vi "GetHighPrioritySensors.vi"   [LabVIEW 2019]
doc: "All high priority sensor reads and safety interlock calculations should be placed in this VI."
uses:
  sensors.vi
  dsdata.vi
  <vilib>/Rock Robotics/WPI/DriverStation/WPI_DriverStationRobotMode2.ctl
  outputs.vi
  refnums.vi
  GRNF_CTREMotor.vi
  <vilib>/Rock Robotics/WPI/ThirdParty/Phoenix-LabVIEW/Motor Controller/Get/CTRE_Phoenix_MotorController_GetSelectedSensorData.vi
  dscommands.vi
  GRNF_DIC.vi
types:
  T1 = typedef "WPI_DriverStationRobotMode2.ctl" = enum16{"Autonomous Disabled", "Autonomous Enabled", "Teleop Disabled", "Teleop Enabled", "Disconnected", "Finish", "Test Disabled", "Test Enabled", "Emergency Stopped"}
  T2 = enum16{"Low Gear", "High Gear", "Transiting", "Unknown", "Force Low Gear"}
  T3 = typedef "WPI_CounterDevRef.ctl" = cluster{"DevStatus":errorcluster, "CntIndex":T4}
  T4 = typedef "FPGA_CounterCtrSystemIndex.ctl" = enum8{"Ctr 0", "Ctr 1", "Ctr 2", "Ctr 3", "Ctr 4", "Ctr 5", "Ctr 6", "Ctr 7", "Invalid"}
  T5 = typedef "WPI_MotorControlDeviceRef.ctl" = cluster{"DeviceStatus":errorcluster, "Type":T6, "PWM":cluster{"PWM Channel":T7, "DeadBand":T8}, "CAN":cluster{"Device Number":u8, "SetOutput VI Ref":variant, "GetOutput VI Ref":variant, "Enable VI Ref":variant, "Disable VI Ref":variant, "Data":variant}, "Invert":bool, "DIO PWM":cluster{"PWM \"Enable\" Channel":T7, "DIOChannel":T9, "PWM Rate":dbl}}
  T6 = typedef "WPI_MotorControlType.ctl" = enum16{"PWM", "CAN", "DIO PWM"}
  T7 = typedef "FPGA_DIOPWMChannel.ctl" = enum8{"PWM 0", "PWM 1", "PWM 2", "PWM 3", "PWM 4", "PWM 5", "PWM 6", "PWM 7", "PWM 8", "PWM 9", "PWM MXP 0", "PWM MXP 1", "PWM MXP 2", "PWM MXP 3", "PWM MXP 4", "PWM MXP 5", "PWM MXP 6", "PWM MXP 7", "PWM MXP 8", "PWM MXP 9", "Invalid"}
  T8 = typedef "WPI_PWMDeadband.ctl" = cluster{"Name":string, "maxPositivePwm":i32, "minPositivePwm":i32, "centerPwm":i32, "maxNegativePwm":i32, "minNegativePwm":i32, "angularRange":u16}
  T9 = typedef "FPGA_DIOChannel.ctl" = enum8{"DIO 0", "DIO 1", "DIO 2", "DIO 3", "DIO 4", "DIO 5", "DIO 6", "DIO 7", "DIO 8", "DIO 9", "DIO MXP 0", "DIO MXP 1", "DIO MXP 2", "DIO MXP 3", "DIO MXP 4", "DIO MXP 5", "DIO MXP 6", "DIO MXP 7", "DIO MXP 8", "DIO MXP 9", "DIO MXP 10", "DIO MXP 11", "DIO MXP 12", "DIO MXP 13", "DIO MXP 14", "DIO MXP 15", "SPI Port CS1", "SPI Port CS2", "SPI Port CS3", "SPI Port MISO", "SPI Port MOSI", "Invalid"}
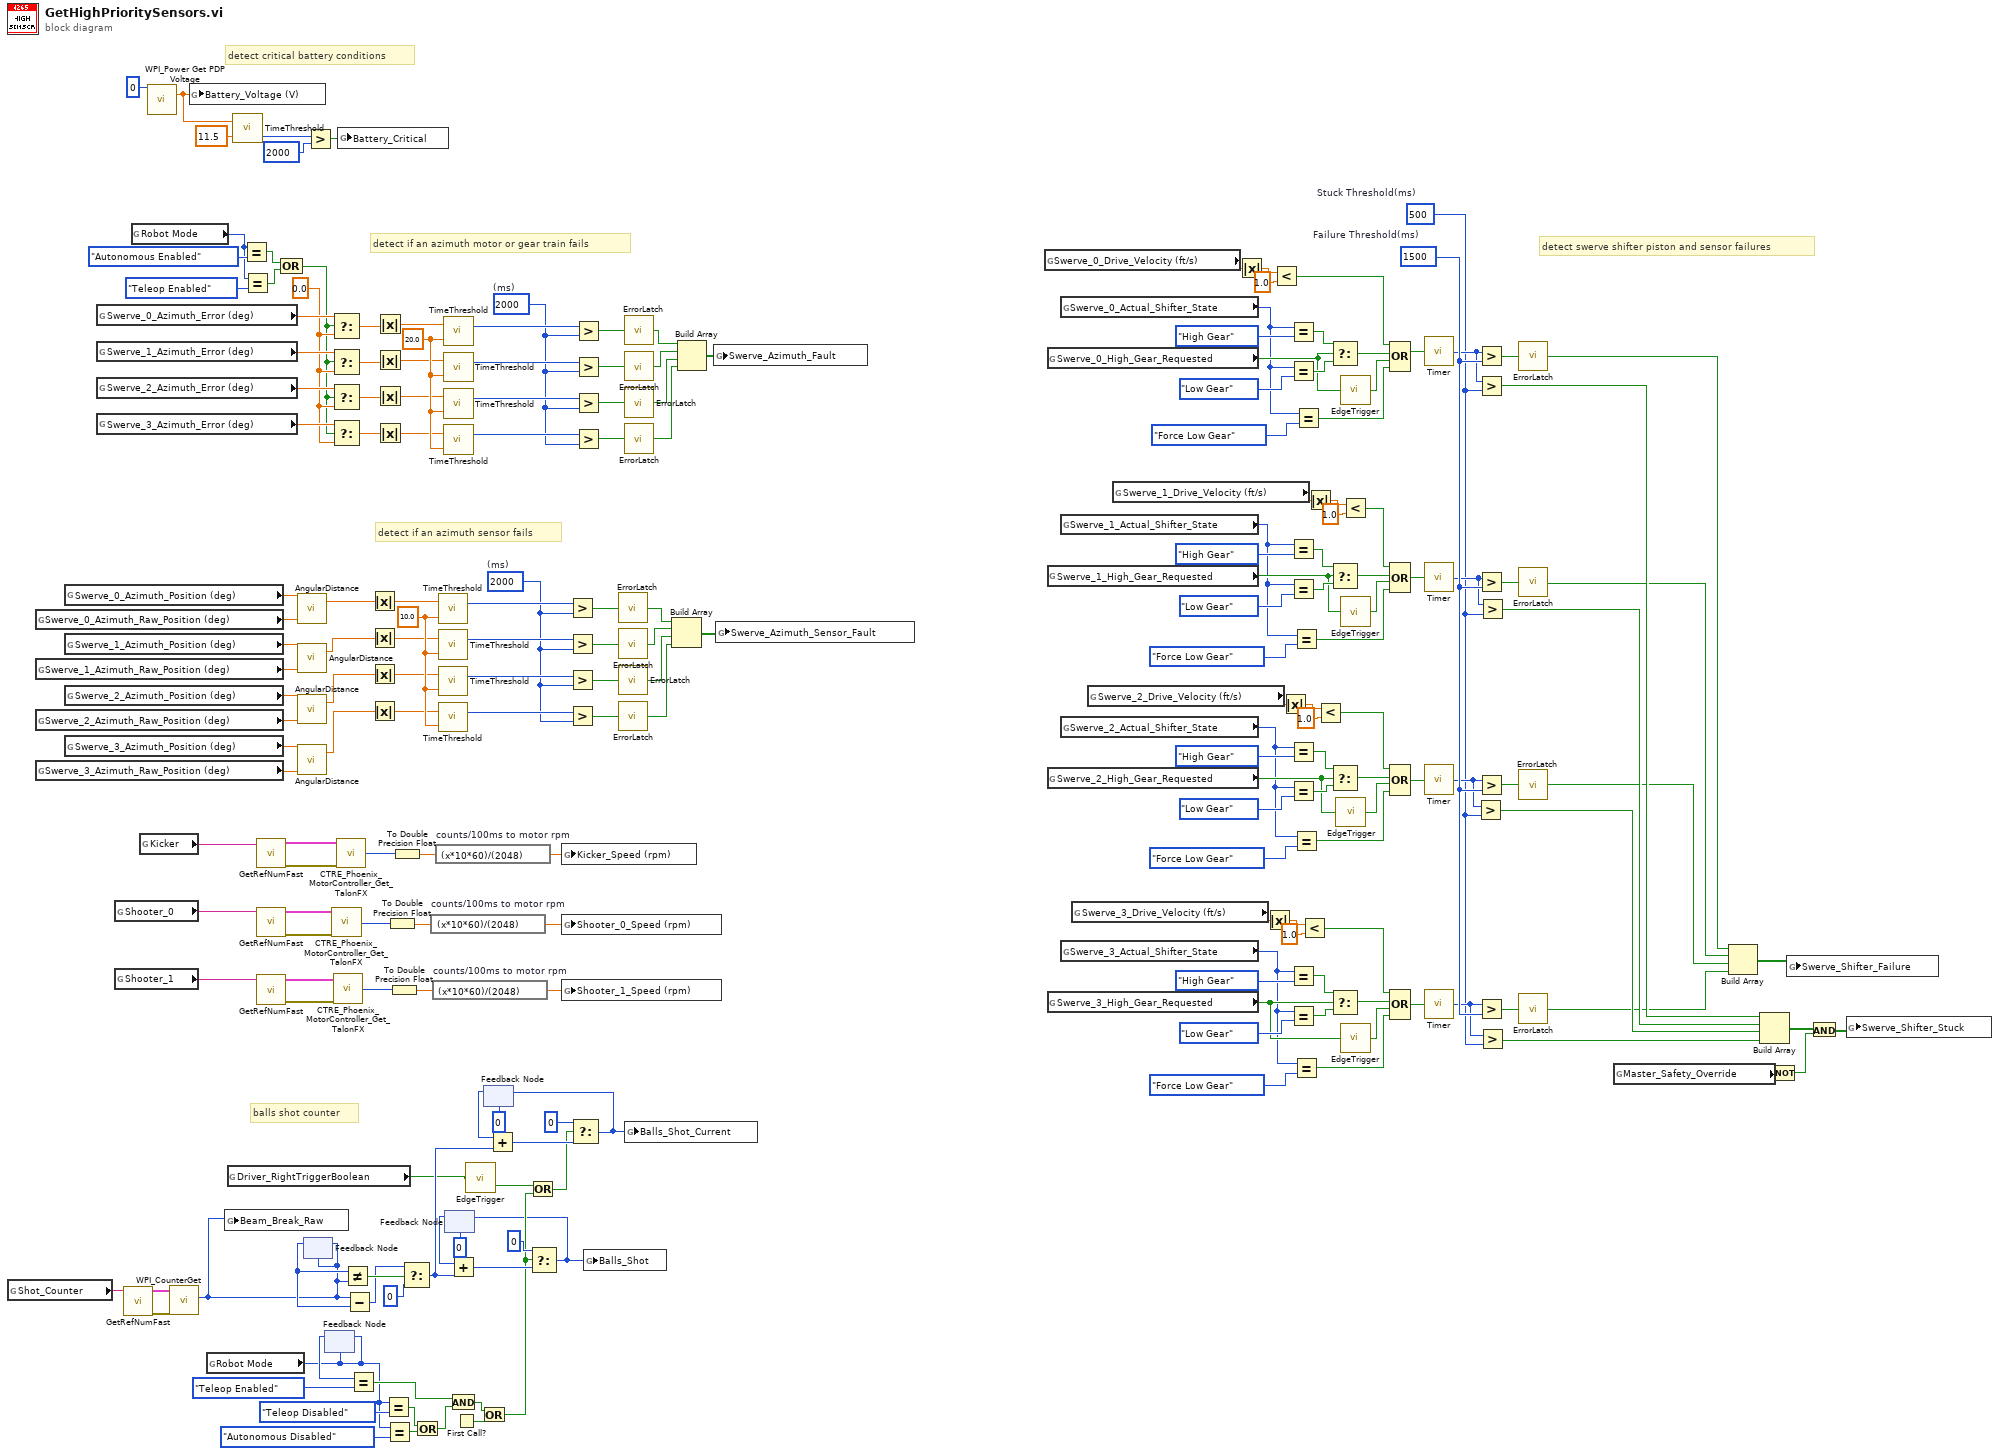
[diagram p0: block diagram]
diagram:
  w99 = u32 500  # Stuck Threshold(ms)
  w124 = u32 2000  # (ms)
  w123 = 10.0 ("Threshold")
  w147 = u32 1500  # Failure Threshold(ms)
  w173 = 0.0
  w196 = u32 2000  # (ms)
  w195 = 20.0 ("Threshold")
  # "balls shot counter"
  # "detect if an azimuth sensor fails"
  # "detect critical battery conditions"
  # "detect swerve shifter piston and sensor failures"
  # "detect if an azimuth motor or gear train fails"
  n1 = global read "refnums.vi" "Shot_Counter"() -> (w15:string)
  n2 = global read "sensors.vi" "Swerve_0_Azimuth_Raw_Position (deg)"() -> (w129:dbl)
  n3 = global read "sensors.vi" "Swerve_1_Azimuth_Raw_Position (deg)"() -> (w108:dbl)
  n4 = global read "sensors.vi" "Swerve_2_Azimuth_Raw_Position (deg)"() -> (w106:dbl)
  n5 = global read "sensors.vi" "Swerve_3_Azimuth_Raw_Position (deg)"() -> (w104:dbl)
  n6 = global read "sensors.vi" "Swerve_0_Azimuth_Position (deg)"() -> (w130:dbl)
  n7 = global read "sensors.vi" "Swerve_1_Azimuth_Position (deg)"() -> (w109:dbl)
  n8 = global read "sensors.vi" "Swerve_2_Azimuth_Position (deg)"() -> (w107:dbl)
  n9 = global read "sensors.vi" "Swerve_3_Azimuth_Position (deg)"() -> (w105:dbl)
  n10 = global read "outputs.vi" "Swerve_0_Azimuth_Error (deg)"() -> (w177:dbl)
  n11 = global read "outputs.vi" "Swerve_1_Azimuth_Error (deg)"() -> (w176:dbl)
  n12 = global read "outputs.vi" "Swerve_2_Azimuth_Error (deg)"() -> (w175:dbl)
  n13 = global read "outputs.vi" "Swerve_3_Azimuth_Error (deg)"() -> (w174:dbl)
  n14 = global read "refnums.vi" "Shooter_0"() -> (w63:string)
  n15 = global read "refnums.vi" "Shooter_1"() -> (w62:string)
  n16 = call-poly "GetRefNumFast.vi"("RefNum Name"=w15) -> ("Error"=w16:errorcluster, "Device Reference"=w17:T3)  [unwired: 5 in]
  n17 = global read "dsdata.vi" "Robot Mode"() -> (w188:T1)
  n18 = global read "refnums.vi" "Kicker"() -> (w64:string)
  n19 = call <vilib>:"WPI_Power Get PDP Voltage.vi"("Power Distribution Panel (0)"=u8 0) -> ("voltage (V)"=w205:dbl)  [unwired: 13 in, 1 out]
  n20 = call <vilib>:"WPI_CounterGet.vi"("error in (no error)"=w16, "CounterDevRef in"=w17) -> ("Value"=w9:i32)  [unwired: 4 in, 5 out]
  n21 = global write "sensors.vi" "Battery_Voltage (V)"(w205) -> ()
  n22 = global read "dsdata.vi" "Robot Mode"() -> (w12:T1)
  n23 = global write "sensors.vi" "Beam_Break_Raw"(w9) -> ()
  n24 = global read "dscommands.vi" "Driver_RightTriggerBoolean"() -> (w13:bool)
  n25 = call "TimeThreshold.vi"("Threshold"=11.5, "Current Value"=w205) -> ("Time Below Threshold (ms)"=w203:u32)  [unwired: 1 out]
  n26 = Equal?(x=w188, y=WPI_DriverStationRobotMode2."Autonomous Enabled") -> (x = y?=w187:bool)
  n27 = Equal?(x=w188, y=WPI_DriverStationRobotMode2."Teleop Enabled") -> (x = y?=w186:bool)
  n28 = call-poly "GetRefNumFast.vi"("RefNum Name"=w64) -> ("Error"=w55:errorcluster, "Device Reference"=w56:T5)  [unwired: 5 in]
  n29 = call-poly "GetRefNumFast.vi"("RefNum Name"=w63) -> ("Error"=w47:errorcluster, "Device Reference"=w48:T5)  [unwired: 5 in]
  n30 = call-poly "GetRefNumFast.vi"("RefNum Name"=w62) -> ("Error"=w45:errorcluster, "Device Reference"=w46:T5)  [unwired: 5 in]
  n31 = Compound Arithmetic op=OR(w187, w186) -> (w168:bool)
  n32 = call "AngularDistance.vi"("Goal Angle (deg) [0,360]"=w129, "Current Angle (deg) [-Inf,+Inf]"=w130) -> ("Signed Angular Distance (deg) [-180,+180]"=w61:dbl)  [unwired: 1 out]
  n33 = call "AngularDistance.vi"("Goal Angle (deg) [0,360]"=w108, "Current Angle (deg) [-Inf,+Inf]"=w109) -> ("Signed Angular Distance (deg) [-180,+180]"=w60:dbl)  [unwired: 1 out]
  n34 = call "AngularDistance.vi"("Goal Angle (deg) [0,360]"=w106, "Current Angle (deg) [-Inf,+Inf]"=w107) -> ("Signed Angular Distance (deg) [-180,+180]"=w59:dbl)  [unwired: 1 out]
  n35 = call "AngularDistance.vi"("Goal Angle (deg) [0,360]"=w104, "Current Angle (deg) [-Inf,+Inf]"=w105) -> ("Signed Angular Distance (deg) [-180,+180]"=w58:dbl)  [unwired: 1 out]
  n36 = feedback #1(w9) -> (w42:i32)
  n37 = feedback-in #1(w9) -> ()
  n38 = Greater?(x=w203, y=u32 2000) -> (0:w201:bool)
  n39 = feedback #2(w12) -> (w32:T1)
  n40 = feedback-in #2(w12) -> ()
  n41 = Select(t=w177, s=w168, f=w173) -> (s? t:f=w172:dbl)
  n42 = Select(t=w176, s=w168, f=w173) -> (s? t:f=w171:dbl)
  n43 = Select(t=w175, s=w168, f=w173) -> (s? t:f=w170:dbl)
  n44 = Select(t=w174, s=w168, f=w173) -> (s? t:f=w169:dbl)
  n45 = call-poly <vilib>:"CTRE_Phoenix_MotorController_Get_TalonFX.vi"("PhoenixMotorControlDevRef"=w48, "error in"=w47) -> ("Velocity (Raw Sensor Units per 100 ms)"=w51:i32)  [unwired: 10 in, 3 out]
  n46 = call-poly <vilib>:"CTRE_Phoenix_MotorController_Get_TalonFX.vi"("PhoenixMotorControlDevRef"=w46, "error in"=w45) -> ("Velocity (Raw Sensor Units per 100 ms)"=w49:i32)  [unwired: 10 in, 3 out]
  n47 = call-poly <vilib>:"CTRE_Phoenix_MotorController_Get_TalonFX.vi"("PhoenixMotorControlDevRef"=w56, "error in"=w55) -> ("Velocity (Raw Sensor Units per 100 ms)"=w53:i32)  [unwired: 10 in, 3 out]
  n48 = global write "sensors.vi" "Battery_Critical"(w201) -> ()
  n49 = Not Equal?(x=w42, y=w9) -> (x != y?=w41:bool)
  n50 = Subtract(x=w9, y=w42) -> (x-y=w40:i32)
  n51 = Equal?(x=w32, y=WPI_DriverStationRobotMode2."Teleop Enabled") -> (x = y?=w31:bool)
  n52 = Absolute Value(x=w61) -> (abs(x)=w122:dbl)
  n53 = Absolute Value(x=w60) -> (abs(x)=w121:dbl)
  n54 = Absolute Value(x=w59) -> (abs(x)=w120:dbl)
  n55 = Absolute Value(x=w58) -> (abs(x)=w119:dbl)
  n56 = Absolute Value(x=w172) -> (abs(x)=w194:dbl)
  n57 = Absolute Value(x=w171) -> (abs(x)=w193:dbl)
  n58 = Absolute Value(x=w170) -> (abs(x)=w192:dbl)
  n59 = Absolute Value(x=w169) -> (abs(x)=w191:dbl)
  n60 = Equal?(x=w12, y=WPI_DriverStationRobotMode2."Teleop Disabled") -> (x = y?=w22:bool)
  n61 = Equal?(x=w12, y=WPI_DriverStationRobotMode2."Autonomous Disabled") -> (x = y?=w23:bool)
  n62 = To Double Precision Float(number=w51) -> (double precision float=w52:dbl)
  n63 = To Double Precision Float(number=w49) -> (double precision float=w50:dbl)
  n64 = To Double Precision Float(number=w53) -> (double precision float=w57:dbl)
  n65 = Select(t=w40, s=w41, f=0) -> (s? t:f=w26:i32)
  n66 = Or(x=w22, y=w23) -> (x .or. y?=w21:bool)
  n67 = expression code="(x*10*60)/(2048)" "counts/100ms to motor rpm"(w52) -> (w44:dbl)
  n68 = expression code="(x*10*60)/(2048)" "counts/100ms to motor rpm"(w50) -> (w43:dbl)
  n69 = expression code="(x*10*60)/(2048)" "counts/100ms to motor rpm"(w57) -> (w54:dbl)
  n70 = call "TimeThreshold.vi"("Threshold"=w123, "Current Value"=w122) -> ("Time Above Threshold (ms)"=w128:u32)  [unwired: 1 out]
  n71 = call "TimeThreshold.vi"("Threshold"=w123, "Current Value"=w121) -> ("Time Above Threshold (ms)"=w127:u32)  [unwired: 1 out]
  n72 = call "TimeThreshold.vi"("Threshold"=w123, "Current Value"=w120) -> ("Time Above Threshold (ms)"=w126:u32)  [unwired: 1 out]
  n73 = call "TimeThreshold.vi"("Threshold"=w123, "Current Value"=w119) -> ("Time Above Threshold (ms)"=w125:u32)  [unwired: 1 out]
  n74 = call "TimeThreshold.vi"("Threshold"=w195, "Current Value"=w194) -> ("Time Above Threshold (ms)"=w200:u32)  [unwired: 1 out]
  n75 = call "TimeThreshold.vi"("Threshold"=w195, "Current Value"=w193) -> ("Time Above Threshold (ms)"=w199:u32)  [unwired: 1 out]
  n76 = call "TimeThreshold.vi"("Threshold"=w195, "Current Value"=w192) -> ("Time Above Threshold (ms)"=w198:u32)  [unwired: 1 out]
  n77 = call "TimeThreshold.vi"("Threshold"=w195, "Current Value"=w191) -> ("Time Above Threshold (ms)"=w197:u32)  [unwired: 1 out]
  n78 = feedback #3(0) -> (w38:i32)
  n79 = Add(x=w38, y=w26) -> (x+y=w36:i32)
  n80 = And(x=w31, y=w21) -> (x .and. y?=w19:bool)
  n81 = First Call?() -> (First Call?: T/F=w20:bool)
  n82 = call "EdgeTrigger.vi"("Input Signal"=w13) -> ("Falling Edge Trigger"=w14:bool)  [unwired: 2 out]
  n83 = Or(x=w19, y=w20) -> (x .or. y?=w18:bool)
  n84 = feedback #4(0) -> (w28:i32)
  n85 = Add(x=w28, y=w26) -> (x+y=w27:i32)
  n86 = Or(x=w14, y=w18) -> (x .or. y?=w25:bool)
  n87 = Select(t=0, s=w18, f=w36) -> (s? t:f=w11:i32)
  n88 = feedback-in #3(w11) -> ()
  n89 = global write "sensors.vi" "Kicker_Speed (rpm)"(w54) -> ()
  n90 = global write "sensors.vi" "Shooter_0_Speed (rpm)"(w44) -> ()
  n91 = global write "sensors.vi" "Shooter_1_Speed (rpm)"(w43) -> ()
  n92 = Greater?(x=w128, y=w124) -> (0:w113:bool)
  n93 = Greater?(x=w127, y=w124) -> (0:w112:bool)
  n94 = Greater?(x=w126, y=w124) -> (0:w111:bool)
  n95 = Greater?(x=w125, y=w124) -> (0:w110:bool)
  n96 = Select(t=0, s=w25, f=w27) -> (s? t:f=w10:i32)
  n97 = feedback-in #4(w10) -> ()
  n98 = Greater?(x=w200, y=w196) -> (0:w181:bool)
  n99 = Greater?(x=w199, y=w196) -> (0:w180:bool)
  n100 = Greater?(x=w198, y=w196) -> (0:w179:bool)
  n101 = Greater?(x=w197, y=w196) -> (0:w178:bool)
  n102 = global write "sensors.vi" "Balls_Shot"(w11) -> ()
  n103 = call "ErrorLatch.vi"("Trigger"=w113) -> ("Latched"=w118:bool)
  n104 = call "ErrorLatch.vi"("Trigger"=w112) -> ("Latched"=w117:bool)
  n105 = call "ErrorLatch.vi"("Trigger"=w111) -> ("Latched"=w116:bool)
  n106 = call "ErrorLatch.vi"("Trigger"=w110) -> ("Latched"=w115:bool)
  n107 = call "ErrorLatch.vi"("Trigger"=w181) -> ("Latched"=w77:bool)
  n108 = call "ErrorLatch.vi"("Trigger"=w180) -> ("Latched"=w185:bool)
  n109 = call "ErrorLatch.vi"("Trigger"=w179) -> ("Latched"=w184:bool)
  n110 = call "ErrorLatch.vi"("Trigger"=w178) -> ("Latched"=w183:bool)
  n111 = global write "sensors.vi" "Balls_Shot_Current"(w10) -> ()
  n112 = Build Array(w118, w117, w116, w115) -> (w114:bool[])
  n113 = Build Array(w77, w185, w184, w183) -> (w182:bool[])
  n114 = global write "sensors.vi" "Swerve_Azimuth_Fault"(w182) -> ()
  n115 = global write "sensors.vi" "Swerve_Azimuth_Sensor_Fault"(w114) -> ()
  n116 = global read "sensors.vi" "Swerve_0_Drive_Velocity (ft/s)"() -> (w94:dbl)
  n117 = global read "outputs.vi" "Swerve_0_High_Gear_Requested"() -> (w146:bool)
  n118 = global read "outputs.vi" "Swerve_1_High_Gear_Requested"() -> (w139:bool)
  n119 = global read "outputs.vi" "Swerve_2_High_Gear_Requested"() -> (w136:bool)
  n120 = global read "outputs.vi" "Swerve_3_High_Gear_Requested"() -> (w131:bool)
  n121 = global read "sensors.vi" "Swerve_0_Actual_Shifter_State"() -> (w66:T2)
  n122 = global read "sensors.vi" "Swerve_1_Actual_Shifter_State"() -> (w69:T2)
  n123 = global read "sensors.vi" "Swerve_2_Actual_Shifter_State"() -> (w72:T2)
  n124 = global read "sensors.vi" "Swerve_3_Actual_Shifter_State"() -> (w75:T2)
  n125 = global read "sensors.vi" "Swerve_3_Drive_Velocity (ft/s)"() -> (w82:dbl)
  n126 = global read "sensors.vi" "Swerve_2_Drive_Velocity (ft/s)"() -> (w86:dbl)
  n127 = global read "sensors.vi" "Swerve_1_Drive_Velocity (ft/s)"() -> (w90:dbl)
  n128 = Absolute Value(x=w94) -> (abs(x)=w93:dbl)
  n129 = Absolute Value(x=w82) -> (abs(x)=w81:dbl)
  n130 = Less?(x=w93, y=1.0) -> (x < y?=w91:bool)
  n131 = Absolute Value(x=w86) -> (abs(x)=w85:dbl)
  n132 = Equal?(x=w66, y=T2."High Gear") -> (x = y?=w166:bool)
  n133 = Equal?(x=w66, y=T2."Low Gear") -> (x = y?=w164:bool)
  n134 = Equal?(x=w69, y=T2."High Gear") -> (x = y?=w161:bool)
  n135 = Equal?(x=w69, y=T2."Low Gear") -> (x = y?=w159:bool)
  n136 = Equal?(x=w72, y=T2."High Gear") -> (x = y?=w156:bool)
  n137 = Equal?(x=w72, y=T2."Low Gear") -> (x = y?=w154:bool)
  n138 = Equal?(x=w75, y=T2."High Gear") -> (x = y?=w151:bool)
  n139 = Equal?(x=w75, y=T2."Low Gear") -> (x = y?=w149:bool)
  n140 = Equal?(x=w69, y=T2."Force Low Gear") -> (x = y?=w68:bool)
  n141 = Equal?(x=w72, y=T2."Force Low Gear") -> (x = y?=w71:bool)
  n142 = Equal?(x=w75, y=T2."Force Low Gear") -> (x = y?=w74:bool)
  n143 = Equal?(x=w66, y=T2."Force Low Gear") -> (x = y?=w65:bool)
  n144 = Less?(x=w81, y=1.0) -> (x < y?=w79:bool)
  n145 = Absolute Value(x=w90) -> (abs(x)=w89:dbl)
  n146 = Less?(x=w85, y=1.0) -> (x < y?=w83:bool)
  n147 = Select(t=w166, s=w146, f=w164) -> (s? t:f=w144:bool)
  n148 = Select(t=w161, s=w139, f=w159) -> (s? t:f=w141:bool)
  n149 = Select(t=w156, s=w136, f=w154) -> (s? t:f=w138:bool)
  n150 = Select(t=w151, s=w131, f=w149) -> (s? t:f=w134:bool)
  n151 = call "EdgeTrigger.vi"("Input Signal"=w136) -> ("All Edge Trigger"=w137:bool)  [unwired: 2 out]
  n152 = call "EdgeTrigger.vi"("Input Signal"=w146) -> ("All Edge Trigger"=w145:bool)  [unwired: 2 out]
  n153 = Less?(x=w89, y=1.0) -> (x < y?=w87:bool)
  n154 = call "EdgeTrigger.vi"("Input Signal"=w139) -> ("All Edge Trigger"=w142:bool)  [unwired: 2 out]
  n155 = call "EdgeTrigger.vi"("Input Signal"=w131) -> ("All Edge Trigger"=w132:bool)  [unwired: 2 out]
  n156 = Compound Arithmetic op=OR(w91, w144, w145, w65) -> (w143:bool)
  n157 = Compound Arithmetic op=OR(w87, w141, w142, w68) -> (w140:bool)
  n158 = Compound Arithmetic op=OR(w83, w138, w137, w71) -> (w135:bool)
  n159 = Compound Arithmetic op=OR(w79, w134, w132, w74) -> (w133:bool)
  n160 = call "Timer.vi"("Reset Timer"=w143) -> ("Time (ms)"=w103:u32)
  n161 = call "Timer.vi"("Reset Timer"=w140) -> ("Time (ms)"=w102:u32)
  n162 = call "Timer.vi"("Reset Timer"=w135) -> ("Time (ms)"=w101:u32)
  n163 = call "Timer.vi"("Reset Timer"=w133) -> ("Time (ms)"=w100:u32)
  n164 = Greater?(x=w101, y=w99) -> (0:w3:bool)
  n165 = Greater?(x=w103, y=w147) -> (0:w163:bool)
  n166 = Greater?(x=w103, y=w99) -> (0:w7:bool)
  n167 = Greater?(x=w102, y=w147) -> (0:w158:bool)
  n168 = Greater?(x=w101, y=w147) -> (0:w153:bool)
  n169 = Greater?(x=w100, y=w147) -> (0:w148:bool)
  n170 = Greater?(x=w102, y=w99) -> (0:w5:bool)
  n171 = Greater?(x=w100, y=w99) -> (0:w2:bool)
  n172 = call "ErrorLatch.vi"("Trigger"=w163) -> ("Latched"=w8:bool)
  n173 = call "ErrorLatch.vi"("Trigger"=w158) -> ("Latched"=w6:bool)
  n174 = call "ErrorLatch.vi"("Trigger"=w153) -> ("Latched"=w4:bool)
  n175 = call "ErrorLatch.vi"("Trigger"=w148) -> ("Latched"=w1:bool)
  n176 = global read "dsdata.vi" "Master_Safety_Override"() -> (w98:bool)
  n177 = Build Array(w8, w6, w4, w1) -> (w78:bool[])
  n178 = Build Array(w7, w5, w3, w2) -> (w97:bool[])
  n179 = Not(x=w98) -> (.not. x?=w96:bool)
  n180 = global write "sensors.vi" "Swerve_Shifter_Failure"(w78) -> ()
  n181 = And(x=w97, y=w96) -> (x .and. y?=w95:bool[])
  n182 = global write "sensors.vi" "Swerve_Shifter_Stuck"(w95) -> ()
